vi "Dashboard Main.vi"() -> ()   [LabVIEW 2012]
uses:
  NonDriveDisplayPanel.ctl
  firstRoboticsCode2012/Snake Game/Snake/xyplot.ctl
  TestProject/Dashboard Datatype.ctl
  TestProject/All_Commands.ctl
  TestProject/Cirular Shooter/circular_shooter_commands.ctl
  TestProject/Climber/Climber_Commands.ctl
  TestProject/All_Outputs.ctl
  TestProject/Cirular Shooter/Shooter_Outputs.ctl
  TestProject/Climber/Climber_Outputs.ctl
  TestProject/All_Sensor_Readings.ctl
  TestProject/Climber/climber_sensor_readings.ctl
  TestProject/Cirular Shooter/Shooter_inputs.ctl
  TestProject/Field Drive/Field_Drive_out.ctl
  TestProject/Joystick_Inputs.ctl
  <vilib>/Rock Robotics/WPI/Joystick/WPI_JoystickButtonState.ctl
  <vilib>/Utility/config.llb/Read Key (String).vi
  <vilib>/Utility/config.llb/Read Key (I32).vi
  <vilib>/Utility/config.llb/NI_LVConfig.lvlib
  <vilib>/vision/NI_Vision_Development_Module.lvlib
panel:
  out "Status":T1(ring)
  in  "Force Hide Snake":bool
  out "direction1":dbl
  in  "Done":bool
  in  "Difficulty":dbl(ring)=15.0 items=["Applications Engineer"=15.0, "Insane"=30.0, "Advanced"=50.0, "Intermediate"=85.0, "Noobie"=125.0]
  in  "Max Apples":i32=10
  out "Score 1":i32
  out "XY Graph":cluster{i32[], i32[]}[](graph)=[{[1000, 990, 980, 970, 960, 950, 940, 930, 920, 910, 900, 890, 880, 870, 860, 850, 840, 830, 820, 810, 800, 790, 780, 770, 760, 750, 740, 730, 720, 710, 700, 690, 680, 670, 660, 650], [500, 500, 500, 500, 500, 500, 500, 500, 500, 500, 500, 500, 500, 500, 500, 500, 500, 500, 500, 500, 500, 500, 500, 500, 500, 500, 500, 500, 500, 500, 500, 500, 500, 500, 500, 500]}, {[-10, 0, 10, 20, 30, 40, 50, 60, 70, 80, 90, 100, 110, 120, 130, 140, 150, 160, 170, 180, 190, 200, 210, 220, 230, 240, 250, 260, 270, 280, 290, 300, 310, 320, 330, 340], [500, 500, 500, 500, 500, 500, 500, 500, 500, 500, 500, 500, 500, 500, 500, 500, 500, 500, 500, 500, 500, 500, 500, 500, 500, 500, 500, 500, 500, 500, 500, 500, 500, 500, 500, 500]}, {[927, 615, 797, 523, 657, 721, 657, 632, 338, 606], [396, 821, 872, 400, 891, 885, 928, 521, 351, 556]}] caption="449"
  out "Score 2":i32
  out "direction2":dbl=2.0
  in  "Add To Score":bool=TRUE
  out "Mechanism Display":T2 {"Current Shooter VBus" scale=0.0..1.0; "Shooter Angle" scale=-10.0..40.0}
  out "Drive Slow Mode":bool
  in  "Running w/ Camera?":bool=TRUE
  out "Camera Image":T3(plugin-control)
  out "Master Caution\nYou mess with the panda,\nsomebody gonna get hurt\nreal bad":bool
  out "Right Joystick":cluster{dbl[], dbl[]}(graph)
  out "Left Joystick":cluster{dbl[], dbl[]}(graph)
  out "BRight":dbl(slide) scale=0.0..1.0
  out "BLeft":dbl(slide) scale=0.0..1.0
  out "FRight":dbl(slide) scale=0.0..1.0
  out "FLeft":dbl(slide) scale=0.0..1.0
  out "Battery Value":dbl(slide) scale=0.0..14.0 scale format="%#_2e"
  out "Battery":sgl(graph)
  out "Mode":T4(ring)=enum."Auto Disabled"
  out "Camera IP":string
  out "Robot IP":string
  # "Wheel Power Requested"
  # "Robot IP:"
  # "Front"
  # "Back"
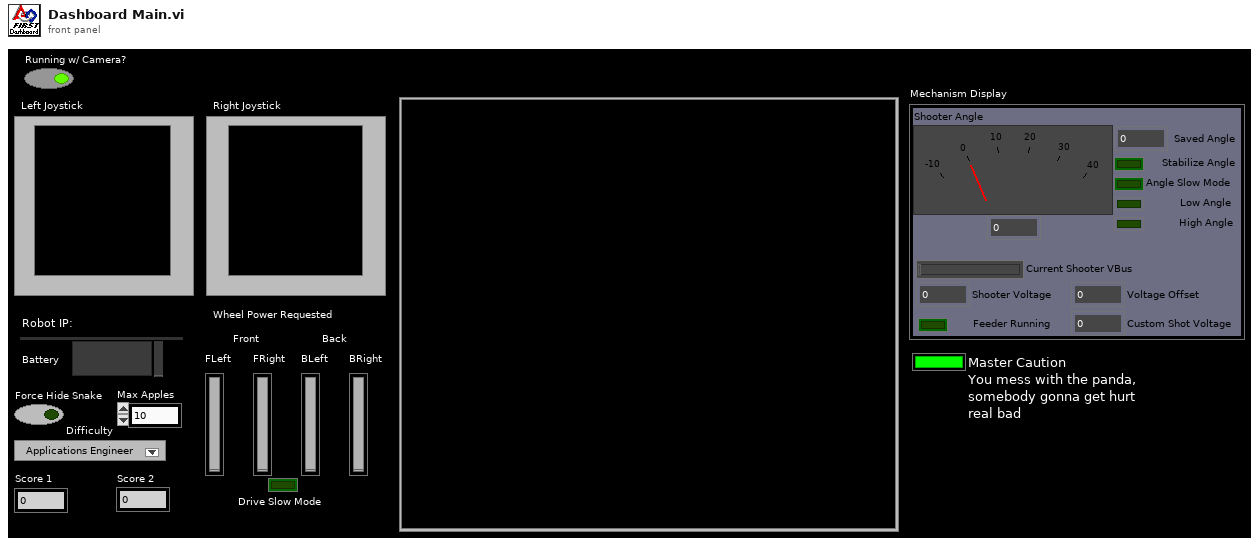
[diagram p1: front panel]
types:
  T1 = enum8{"Disconnected", "E-Stop", "Disabled", "Enabled"}
  T2 = typedef "NonDriveDisplayPanel.ctl" = cluster{"Shooter Angle":dbl, "Current Shooter VBus":dbl, "Shooter Voltage":dbl, "Feeder Running":bool, "Saved Angle":dbl, "Stabilize Angle":bool, "Voltage Offset":dbl, "Custom Shot Voltage":dbl, "Angle Slow Mode":bool, "Low Angle ":bool, "High Angle":bool}
  T3 = typedef "IMAQ Image.ctl" = refnum<image>
  T4 = enum8{"Tele-Op Disabled", "Tele-Op Enabled", "Auto Disabled", "Auto Enabled", "Test Disabled", "Test Enabled", ""}
  T5 = typedef "Image Type" = u32
  T6 = typedef "Dashboard Datatype.ctl" = cluster{"All Driver Commands":T7, "All_Outputs":T10, "All_Sensor_Readings":T13, "Joystick_Inputs ":T17}
  T7 = typedef "All_Commands.ctl" = cluster{"Circular Shooter Commands":T8, "Drive Command Inputs":cluster{"Strafe":dbl, "Forward/Backward":dbl, "Rotation":dbl, "Drive Slow Toggle":bool}, "Climber_Commands":T9}
  T8 = typedef "circular_shooter_commands.ctl" = cluster{"Shoot?":bool, "Angle Change":dbl, "Close Shot":bool, "Far Shot":bool, "Stabilize Angle ":bool, "Offset":dbl, "Custom Shot":bool, "Custom Shot Voltage":dbl, "Low Angle":bool, "High Angle":bool, "Angle Slow Mode":bool, "Dejam":bool, "Save Angle":bool, "Saved Preset Angle":bool}
  T9 = typedef "Climber_Commands.ctl" = cluster{"Assist":dbl}
  T10 = typedef "All_Outputs.ctl" = cluster{"Drive Outputs":cluster{"Front Left\nSpeed":dbl, "Back Left\nSpeed":dbl, "Front Right\nSpeed":dbl, "Back Right\nSpeed":dbl}, "Shooter_Outputs":T11, "Climber_Outputs":T12}
  T11 = typedef "Shooter_Outputs.ctl" = cluster{"Feeder_Motor_Voltage":dbl, "Output Voltage":dbl, "Overloaded":bool, "Variable_Angle_Voltage":dbl, "Saved Angle":dbl}
  T12 = typedef "Climber_Outputs.ctl" = cluster{"Assist Voltage":dbl}
  T13 = typedef "All_Sensor_Readings.ctl" = cluster{"Climber Inputs":T14, "Drive Sensor Readings":cluster{"Front Left\nSpeed":dbl, "Back Left\nSpeed":dbl, "Front Right\nSpeed":dbl, "Back Right\nSpeed":dbl}, "Shooter_Inputs":T15, "Field_Drive_Out\n":T16}
  T14 = typedef "climber_sensor_readings.ctl" = cluster{"Top Left Switch":bool, "Bottom Left Switch":bool, "Top Right Switch":bool, "Bottom Right Switch":bool}
  T15 = typedef "Shooter_inputs.ctl" = cluster{"Bus Voltage":dbl, "Output Percent VBus":dbl, "Shooter Elevation Angle":dbl, "FeederPosition":bool}
  T16 = typedef "Field_Drive_out.ctl" = cluster{"XPos":dbl, "Ypos":dbl, "XVel":dbl, "YVel":dbl, "Heading":dbl, "AngularVel":dbl, "F_XPos":dbl, "F_Ypos":dbl, "F_Angle":dbl}
  T17 = typedef "Joystick_Inputs.ctl" = cluster{"Joystick 1":cluster{"Axes":cluster{"axis 1 (x)":dbl, "axis 2 (y)":dbl, "axis 3 (throttle)":dbl, "axis 4":dbl, "axis 5":dbl, "axis 6":dbl}, "Buttons":T18}, "Joystick 2":cluster{"Axes":cluster{"axis 1 (x)":dbl, "axis 2 (y)":dbl, "axis 3 (throttle)":dbl, "axis 4":dbl, "axis 5":dbl, "axis 6":dbl}, "Buttons":T18}, "Joystick 3":cluster{"Axes":cluster{"axis 1 (x)":dbl, "axis 2 (y)":dbl, "axis 3 (throttle)":dbl, "axis 4":dbl, "axis 5":dbl, "axis 6":dbl}, "Buttons":T18}, "Joystick 4":cluster{"Axes":cluster{"axis 1 (x)":dbl, "axis 2 (y)":dbl, "axis 3 (throttle)":dbl, "axis 4":dbl, "axis 5":dbl, "axis 6":dbl}, "Buttons":T18}}
  T18 = typedef "WPI_JoystickButtonState.ctl" = cluster{"Button 1":bool, "Button 2":bool, "Button 3":bool, "Button 4":bool, "Button 5":bool, "Button 6":bool, "Button 7":bool, "Button 8":bool, "Button 9":bool, "Button 10":bool, "Button 11":bool, "Button 12":bool}
  T19 = cluster{"Competition mode":bool, "Robot Link":bool, "Autonomous":bool, "Enabled":bool, "E-Stop":bool, "Simulated":bool, "TestMode":bool, "Docked Window":bool}
  T20 = typedef "LVRectTypeDef.ctl" = cluster{"Left":i16, "Top":i16, "Right":i16, "Bottom":i16}
  T21 = typedef "NI_LVConfig.lvlib/Config Data RefNum.ctl" = refnum<k1>
  T22 = typedef "xyplot.ctl" = cluster{"X":i32[], "Y":i32[]}
  T23 = typedef "eventvkey.ctl" = enum16{"ASCII", "Enter", "Return", "Shift", "Ctrl", "Alt", "Cmd", "Opt", "Caps", "NumLock", "Clear", "Break", "Up", "Down", "Left", "Right", "Insert", "Delete", "Home", "End", "PageUp", "PageDown", "Escape", "Help", "Pause", "ScrollLock", "F1", "F2", "F3", "F4", "F5", "F6", "F7", "F8", "F9", "F10", "F11", "F12", "F13", "F14", "F15", "F16", "F17", "F18", "F19", "F20", "F21", "F22", "F23", "F24", "Play", "VolumeUp", "VolumeDown", "Mute", "Two Byte Char"}
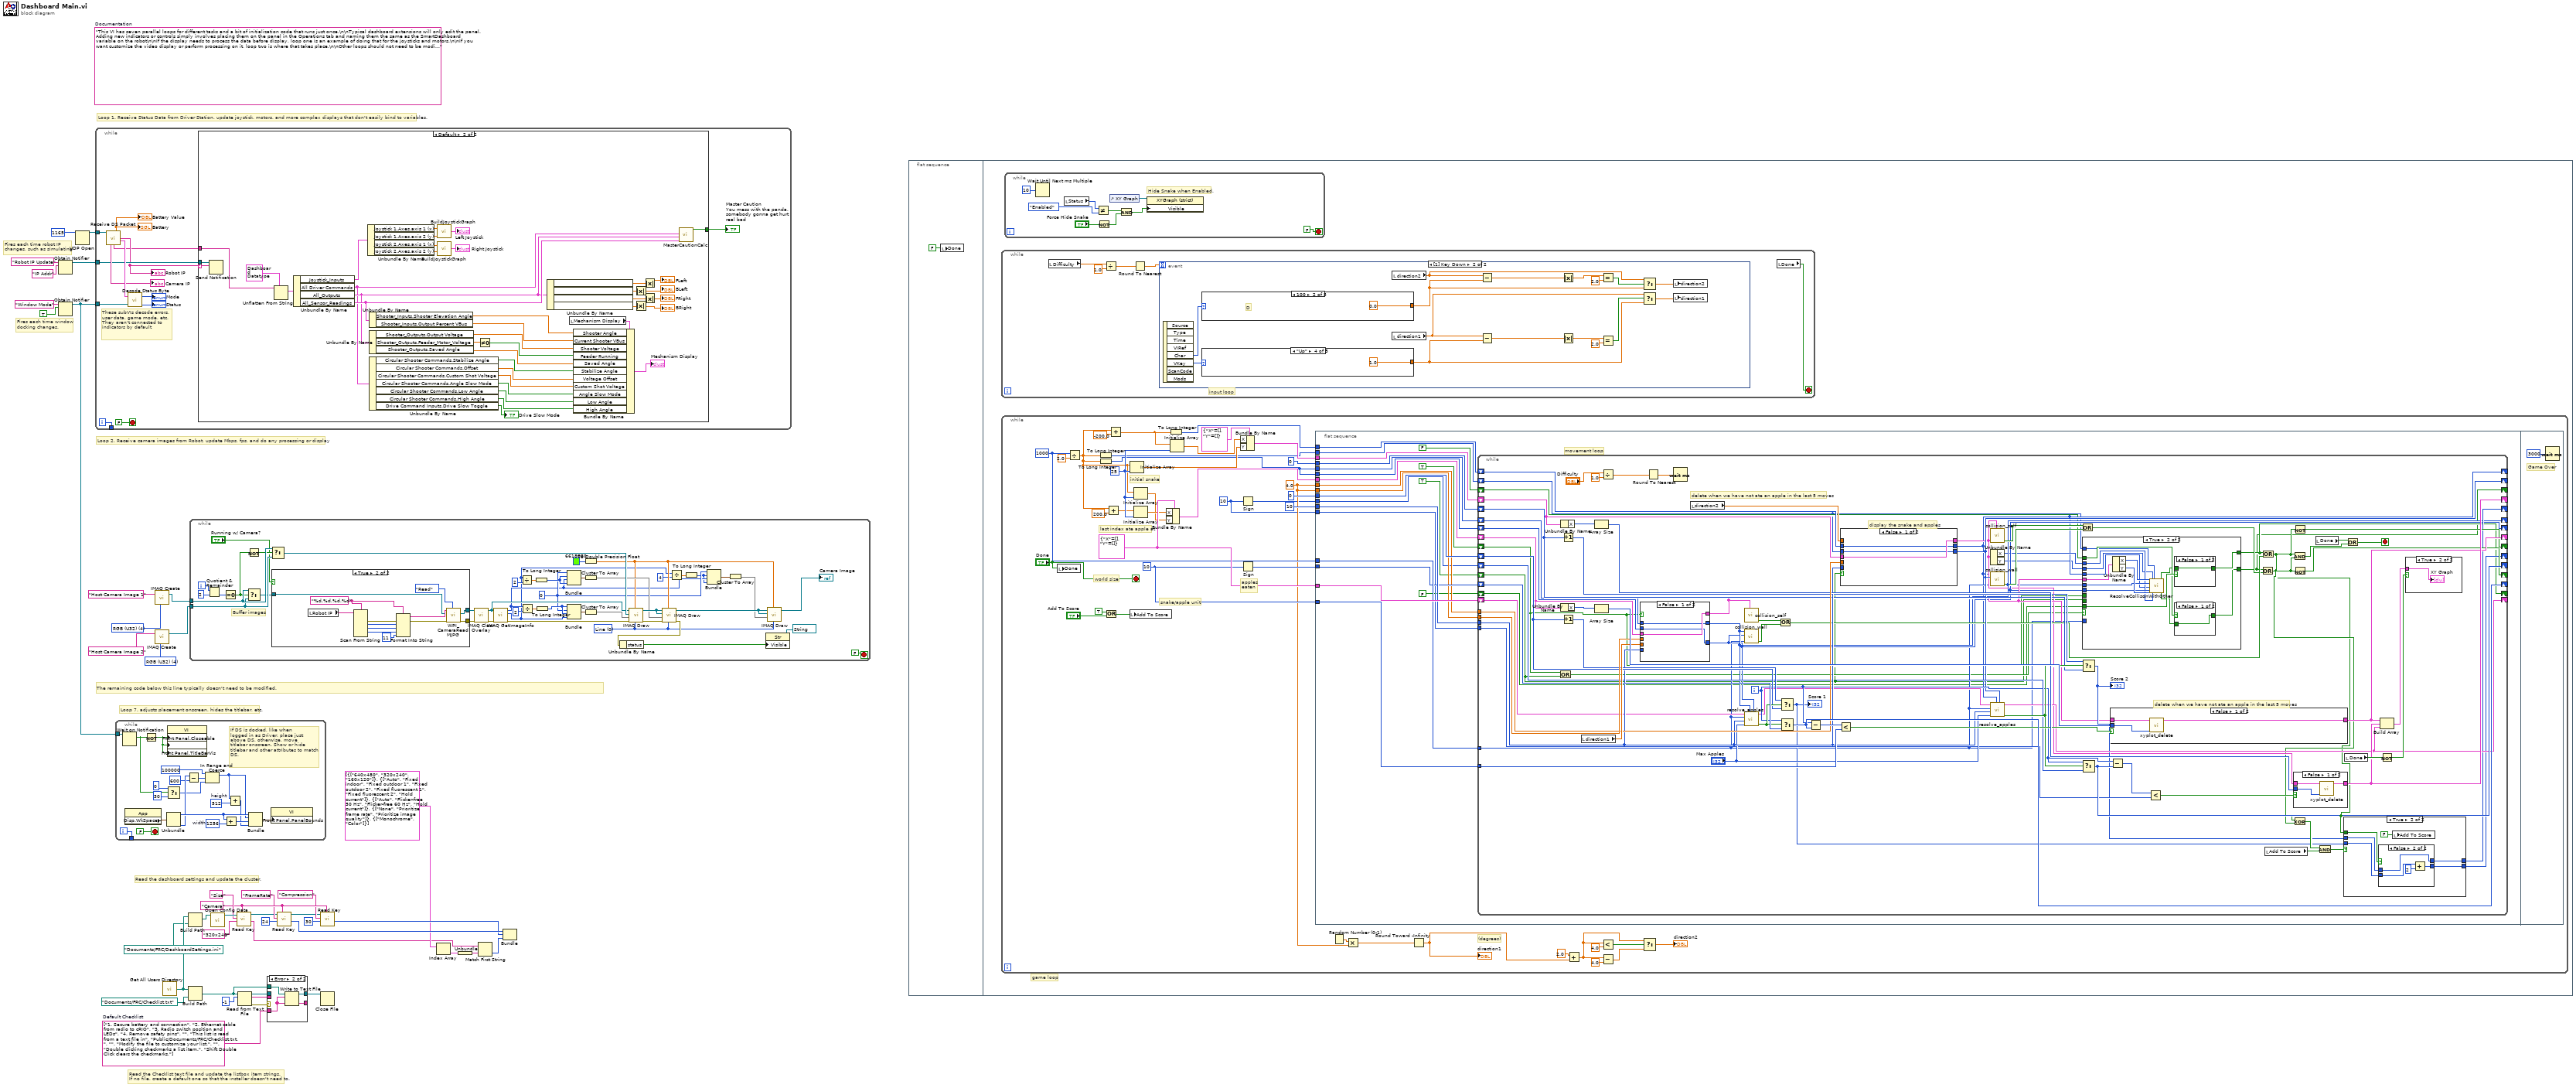
[diagram p0: block diagram]
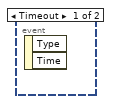
[diagram p2: hidden frame]
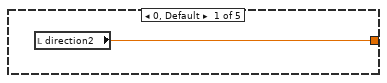
[diagram p3: hidden frame]
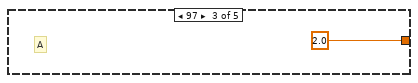
[diagram p4: hidden frame]
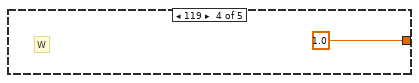
[diagram p5: hidden frame]
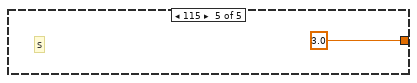
[diagram p6: hidden frame]
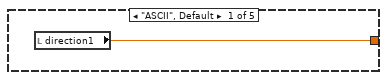
[diagram p7: hidden frame]
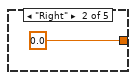
[diagram p8: hidden frame]
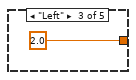
[diagram p9: hidden frame]
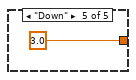
[diagram p10: hidden frame]
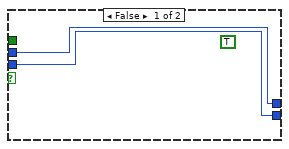
[diagram p16: hidden frame]
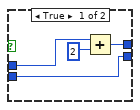
[diagram p17: hidden frame]
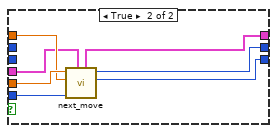
[diagram p18: hidden frame]
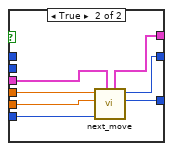
[diagram p19: hidden frame]
diagram:
  (unwired) "320x240"
  w3 = T5 4 items=["Grayscale (U8)", "Grayscale (I16)", "Grayscale (SGL)", "Complex (CSG)", "RGB (U32)", "HSL (U32)", "RGB (U64)", "Grayscale (U16)"] ("Image Type")
  w6 = T5 4 items=["Grayscale (U8)", "Grayscale (I16)", "Grayscale (SGL)", "Complex (CSG)", "RGB (U32)", "HSL (U32)", "RGB (U64)"] ("Image Type")
  w23 = "Camera"
  w29 = string[] ["1. Secure battery and connection", "2. Ethernet cable from radio to cRIO", "3. Radio switch position and LEDs", "4. Remove safety pins", "", "This list is read from a text file in", "Public/Documents/FRC/Checklist.txt.", "", "Modify the file to customize your list.", "", "Double clicking checkmarks a list item.", "Shift Double Click clears the checkmarks."]  # Default Checklist
  (unwired) "This VI has seven parallel loops for different tasks and a bit of initialization code that runs just once.\n\nTypical dashboard extensions will only edit the panel. Adding new indicators or controls simply involves placing them on the panel in the Operations tab and naming them the same as the SmartDashboard variable on the robot\n\nIf the display needs to process the data before display, loop one is an example of doing that for the joysticks and motors.\n\nIf you want customize the video display or perform processing on it, loop two is where that takes place.\n\nOther loops should not need to be modified. They are pretty standard, and document the task they perform."  # Documentation
  # "Fires each time robot IP\nchanges, such as simulating"
  # "Fires each time window\ndocking changes."
  # "Read the Checklist text file and update the listbox item strings.\nIf no file, create a default one so that the installer doesn't need to."
  # "The remaining code below this line typically doesn't need to be modified."
  # "Read the dashboard settings and update the cluster."
  # "Loop 7. adjusts placement onscreen, hides the titlebar, etc."
  # "Loop 1. Receive Status Data from Driver Station, update joystick, motors, and more complex displays that don't easily bind to variables."
  # "Loop 2. Receive camera images from Robot, update Mbps, fps, and do any processing or display"
  n1 = Obtain Notifier(name (unnamed)="Robot IP Update", notification data type="IP Addr" ("name (unnamed)")) -> (notifier out=w38:refnum<notifier>)  [unwired: 2 in, 2 out]
  n2 = Obtain Notifier(name (unnamed)="Window Mode", notification data type=TRUE) -> (notifier out=w33:refnum<notifier>)  [unwired: 2 in, 2 out]
  n3 = UDP Open(11:u16 1165 ("port")) -> (port=w41:refnum<k16>)  [unwired: 2 in, 4 out]
  n4 = while {
    tunnel: w41 -> [w53]
    tunnel: w38 -> [w47]
    tunnel: w33 -> [w51]
    tunnel: [w48] -> _
    i -> [w48]
    stop <- FALSE stop-if-true
    # "These subVIs decode errors, user data, game mode, etc.\nThey aren't connected to indicators by default"
    n5 = call "Receive DS Packet.vi"("Recv Socket"=w53) -> ("Battery"=→"Battery" →"Battery Value":sgl, "Robot IP Address"=w46:string, "Status"=w54:T19, "Camera IP Address"=→"Camera IP":string, "Low Priority User Data"=w43:string)  [unwired: 1 in, 9 out]
    "Robot IP" <- w46
    n6 = call "Decode Status Byte.vi"("Window Mode Notifier"=w51, "Status"=w54) -> ("Status"=→"Status":T1, "Mode"=→"Mode":T4)
    n7 = case shown="Default" w46 {
      selector: w46 -> [_ w94]
      tunnel: w47 -> [_ w95]
      tunnel: [TRUE w77] -> w45
      tunnel: w43 -> [_ w59]
      frame "0.0.0.0" {
        # "Robot not responding, don't poll the variables"
      }
      frame Default {
        n8 = Send Notification(notification=w94, notifier=w95) -> ()  [unwired: 1 in, 2 out]
        n9 = Unflatten From String(type=T6 {"All Driver Commands"={"Circular Shooter Commands"={"Shoot?"=FALSE, "Angle Change"=0.0, "Close Shot"=FALSE, "Far Shot"=FALSE, "Stabilize Angle "=FALSE, "Offset"=0.0, "Custom Shot"=FALSE, "Custom Shot Voltage"=0.0, "Low Angle"=FALSE, "High Angle"=FALSE, "Angle Slow Mode"=FALSE, "Dejam"=FALSE, "Save Angle"=FALSE, "Saved Preset Angle"=FALSE}, "Drive Command Inputs"={"Strafe"=0.0, "Forward/Backward"=0.0, "Rotation"=0.0, "Drive Slow Toggle"=FALSE}, "Climber_Commands"={"Assist"=0.0}}, "All_Outputs"={"Drive Outputs"={"Front Left\nSpeed"=0.0, "Back Left\nSpeed"=0.0, "Front Right\nSpeed"=0.0, "Back Right\nSpeed"=0.0}, "Shooter_Outputs"={"Feeder_Motor_Voltage"=0.0, "Output Voltage"=0.0, "Overloaded"=FALSE, "Variable_Angle_Voltage"=0.0, "Saved Angle"=0.0}, "Climber_Outputs"={"Assist Voltage"=0.0}}, "All_Sensor_Readings"={"Climber Inputs"={"Top Left Switch"=FALSE, "Bottom Left Switch"=FALSE, "Top Right Switch"=FALSE, "Bottom Right Switch"=FALSE}, "Drive Sensor Readings"={"Front Left\nSpeed"=0.0, "Back Left\nSpeed"=0.0, "Front Right\nSpeed"=0.0, "Back Right\nSpeed"=0.0}, "Shooter_Inputs"={"Bus Voltage"=0.0, "Output Percent VBus"=0.0, "Shooter Elevation Angle"=0.0, "FeederPosition"=FALSE}, "Field_Drive_Out\n"={"XPos"=0.0, "Ypos"=0.0, "XVel"=0.0, "YVel"=0.0, "Heading"=0.0, "AngularVel"=0.0, "F_XPos"=0.0, "F_Ypos"=0.0, "F_Angle"=0.0}}, "Joystick_Inputs "={"Joystick 1"={"Axes"={"axis 1 (x)"=0.0, "axis 2 (y)"=0.0, "axis 3 (throttle)"=0.0, "axis 4"=0.0, "axis 5"=0.0, "axis 6"=0.0}, "Buttons"={"Button 1"=FALSE, "Button 2"=FALSE, "Button 3"=FALSE, "Button 4"=FALSE, "Button 5"=FALSE, "Button 6"=FALSE, "Button 7"=FALSE, "Button 8"=FALSE, "Button 9"=FALSE, "Button 10"=FALSE, "Button 11"=FALSE, "Button 12"=FALSE}}, "Joystick 2"={"Axes"={"axis 1 (x)"=0.0, "axis 2 (y)"=0.0, "axis 3 (throttle)"=0.0, "axis 4"=0.0, "axis 5"=0.0, "axis 6"=0.0}, "Buttons"={"Button 1"=FALSE, "Button 2"=FALSE, "Button 3"=FALSE, "Button 4"=FALSE, "Button 5"=FALSE, "Button 6"=FALSE, "Button 7"=FALSE, "Button 8"=FALSE, "Button 9"=FALSE, "Button 10"=FALSE, "Button 11"=FALSE, "Button 12"=FALSE}}, "Joystick 3"={"Axes"={"axis 1 (x)"=0.0, "axis 2 (y)"=0.0, "axis 3 (throttle)"=0.0, "axis 4"=0.0, "axis 5"=0.0, "axis 6"=0.0}, "Buttons"={"Button 1"=FALSE, "Button 2"=FALSE, "Button 3"=FALSE, "Button 4"=FALSE, "Button 5"=FALSE, "Button 6"=FALSE, "Button 7"=FALSE, "Button 8"=FALSE, "Button 9"=FALSE, "Button 10"=FALSE, "Button 11"=FALSE, "Button 12"=FALSE}}, "Joystick 4"={"Axes"={"axis 1 (x)"=0.0, "axis 2 (y)"=0.0, "axis 3 (throttle)"=0.0, "axis 4"=0.0, "axis 5"=0.0, "axis 6"=0.0}, "Buttons"={"Button 1"=FALSE, "Button 2"=FALSE, "Button 3"=FALSE, "Button 4"=FALSE, "Button 5"=FALSE, "Button 6"=FALSE, "Button 7"=FALSE, "Button 8"=FALSE, "Button 9"=FALSE, "Button 10"=FALSE, "Button 11"=FALSE, "Button 12"=FALSE}}}} ("Dashboard Data"), binary string=w59) -> (value=w93:T6)  [unwired: 3 in, 2 out]
        n10 = Unbundle By Name(w93) -> ("Joystick_Inputs"=w84:T17, "All Driver Commands"=w73:T7, "All_Outputs"=w75:T10, "All_Sensor_Readings"=w76:T13)
        n11 = Unbundle By Name(w84) -> ("Joystick 1.Axes.axis 1 (x)"=w81:dbl, "Joystick 1.Axes.axis 2 (y)"=w80:dbl, "Joystick 2.Axes.axis 1 (x)"=w79:dbl, "Joystick 2.Axes.axis 2 (y)"=w78:dbl)
        n12 = Unbundle By Name(w76) -> ("Shooter_Inputs.Shooter Elevation Angle"=w57:dbl, "Shooter_Inputs.Output Percent VBus"=w70:dbl)
        n13 = Unbundle By Name(w75) -> ("Shooter_Outputs.Output Voltage"=w69:dbl, "Shooter_Outputs.Feeder_Motor_Voltage"=w74:dbl, "Shooter_Outputs.Saved Angle"=w67:dbl)
        n14 = Unbundle By Name(w73) -> ("Circular Shooter Commands.Stabilize Angle"=w66:bool, "Circular Shooter Commands.Offset"=w65:dbl, "Circular Shooter Commands.Custom Shot Voltage"=w64:dbl, "Circular Shooter Commands.Angle Slow Mode"=w63:bool, "Circular Shooter Commands.Low Angle"=w61:bool, "Circular Shooter Commands.High Angle"=w60:bool, "Drive Command Inputs.Drive Slow Toggle"=→"Drive Slow Mode":bool)
        n15 = call "BuildJoystickGraph.vi"("YAxis"=w80, "XAxis"=w81) -> ("Left Joystick"=→"Left Joystick":cluster{dbl[], dbl[]})
        n16 = call "BuildJoystickGraph.vi"("YAxis"=w78, "XAxis"=w79) -> ("Left Joystick"=→"Right Joystick":cluster{dbl[], dbl[]})
        n17 = Not Equal To 0?(x=w74) -> (x != 0?=w68:bool)
        n18 = Unbundle By Name(w75) -> ("Drive Outputs.Front Left\nSpeed"=w92:dbl, "Drive Outputs.Back Left\nSpeed"=w91:dbl, "Drive Outputs.Front Right\nSpeed"=w89:dbl, "Drive Outputs.Back Right\nSpeed"=w90:dbl)
        n19 = local read "Mechanism Display"() -> (w71:T2)
        n20 = Bundle By Name(cluster=w71, "Shooter Angle"=w57, "Current Shooter VBus"=w70, "Shooter Voltage"=w69, "Feeder Running"=w68, "Saved Angle"=w67, "Stabilize Angle"=w66, "Voltage Offset"=w65, "Custom Shot Voltage"=w64, "Angle Slow Mode"=w63, "Low Angle"=w61, "High Angle"=w60) -> (→"Mechanism Display":T2)
        n21 = Absolute Value(x=w91) -> (abs(x)=→"BLeft":dbl)
        n22 = Absolute Value(x=w90) -> (abs(x)=→"BRight":dbl)
        n23 = Absolute Value(x=w92) -> (abs(x)=→"FLeft":dbl)
        n24 = Absolute Value(x=w89) -> (abs(x)=→"FRight":dbl)
        n25 = call "MasterCautionCalc.vi"("All_Sensor_Readings"=w76, "All_Outputs"=w75, "All Driver Commands"=w73) -> ("Master Caution"=w77:bool)  [unwired: 8 in]
      }
    }
    "Master Caution\nYou mess with the panda,\nsomebody gonna get hurt\nreal bad" <- w45
  }
  n26 = while {
    tunnel: w33 -> [w114]
    tunnel: [w112] -> _
    i -> [w112]
    stop <- FALSE stop-if-true
    w104 = 1256  # width
    w107 = 512  # height
    # "If DS is docked, like when\nlogged in as Driver, place just\nabove DS, otherwise, move\ntitlebar onscreen. Show or hide\ntitlebar and other attributes to match\nDS."
    n27 = Wait on Notification(notifier=w114) -> (notification=w99:bool)  [unwired: 3 in, 3 out]
    n28 = property class="App"() -> ("Disp.WkSpace"=w110:T20)  [unwired: 2 in, 2 out]
    n29 = Not(x=w99) -> (.not. x?=w113:bool)
    n30 = Unbundle(w110) -> ("Left"=w108:i16, "Bottom"=w105:i16)  [unwired: 2 out]
    n31 = Select(t=0, s=w99, f=30) -> (s? t:f=w98:i32)
    n32 = property class="VI"("Front Panel.Closeable"=w113, "Front Panel.Minimizeable"=w113, "Front Panel.TitleBarVis"=w113) -> ()  [unwired: 2 in, 2 out]
    n33 = Subtract(x=w105, y=600) -> (x-y=w102:i32)
    n34 = In Range and Coerce(upper limit=100000, x=w102, lower limit=w98) -> (coerced(x)=w96:i32)  [unwired: 1 out]
    n35 = Add(x=w108, y=w104) -> (x+y=w109:i32)
    n36 = Add(x=w96, y=w107) -> (x+y=w106:i32)
    n37 = Bundle("Left"=w108, w96, w109, w106) -> (w111:cluster{"Left":i16, i32, i32, i32})  [unwired: 1 out]
    n38 = property class="VI"("Front Panel.PanelBounds"=w111) -> ()  [unwired: 2 in, 2 out]
  }
  n39 = call "IMAQ Create"("Image Name"="Host Camera Image 1", "Image Type"=w6) -> ("New Image"=w2:T3)  [unwired: 2 in, 2 out]
  n40 = call "IMAQ Create"("Image Name"="Host Camera Image 2", "Image Type"=w3) -> ("New Image"=w1:T3)  [unwired: 3 in, 1 out]
  n41 = call "Get All Users Directory.vi"() -> ("All User Path"=w28:path)
  n42 = Build Path(base path=w28, name or relative path=path "Documents/FRC/DashboardSettings.ini") -> (appended path=w27:path)
  n43 = Build Path(base path=w28, name or relative path=path "Documents/FRC/Checklist.txt") -> (appended path=w30:path)
  n44 = while {
    tunnel: w2 -> [w158]
    tunnel: w1 -> [w153]
    i -> [w157]
    stop <- FALSE stop-if-true
    w121 = 0
    w124 = u16 0 items=["Line", "Rectangle", "Oval"] ("Shape to draw")
    # "Buffer images"
    n45 = Quotient & Remainder(x=w157, y=2) -> (floor(x/y)=w155:i32)  [unwired: 1 out]
    n46 = Equal To 0?(x=w155) -> (x = 0?=w154:bool)
    n47 = Not(x=w154) -> (.not. x?=w144:bool)
    n48 = Select(t=w158, s=w154, f=w153) -> (s? t:f=w141:T3)
    n49 = Select(t=w158, s=w144, f=w153) -> (s? t:f=w143:T3)
    n50 = case shown="True" "Running w/ Camera?" {
      tunnel: w141 -> [w169 w172]
      tunnel: [w167 w170] -> w146
      tunnel: [w168 w171] -> w145
      frame False {
        n51 = Current VI's Path() -> (path=w166:path)
        n52 = Strip Path(path=w166) -> (stripped path=w165:path)  [unwired: 1 out]
        n53 = Strip Path(path=w165) -> (stripped path=w160:path)  [unwired: 1 out]
        n54 = Build Path(base path=w160, name or relative path="Vision") -> (appended path=w163:path)
        n55 = Build Path(base path=w163, name or relative path="Field1.jpg") -> (appended path=w161:path)
        n56 = call "IMAQ ReadFile"("File Path"=w161, "Image"=w169) -> ("error out"=w167:errorcluster, "Image Out"=w168:T3)  [unwired: 5 in, 3 out]
      }
      frame True {
        w176 = "%d.%d.%d.%d" ("format string")
        n57 = local read "Robot IP"() -> (w173:string)
        n58 = Scan From String(format string=w176, input string=w173) -> (error out=w179:errorcluster, output 1=w180:i32, output 2=w181:i32, output 3=w182:i32)  [unwired: 2 in, 7 out]
        n59 = Format Into String(format string=w176, error in=w179, w180, w181, w182, 11 ("IP Suffix:")) -> (resulting string=w178:string, error out=w177:errorcluster)  [unwired: 1 in]
        n60 = call <vilib>:"WPI_CameraRead MJPG.vi"("Operation"=enum16{"Read", "Reopen", "Close"}."Read", "error in"=w177, "Image"=w172, "address"=w178) -> ("error out"=w170:errorcluster, "Image Out"=w171:T3)  [unwired: 5 in, 1 out]
      }
    }
    n61 = call "IMAQ Clear Overlay"("error in (no error)"=w146, "Image"=w145) -> ("error out"=w139:errorcluster, "Image Out"=w140:T3)  [unwired: 8 in]
    n62 = call "IMAQ GetImageInfo"("error in (no error)"=w139, "Image"=w140) -> ("error out"=w147:errorcluster, "Y Resolution"=w119:i32, "X Resolution"=w120:i32)  [unwired: 2 in, 5 out]
    n63 = Divide(x=w119, y=2) -> (x/y=w130:dbl)
    n64 = Divide(x=w120, y=2) -> (x/y=w151:dbl)
    n65 = To Long Integer(number=w130) -> (32bit integer=w129:i32)
    n66 = To Long Integer(number=w151) -> (32bit integer=w150:i32)
    n67 = Bundle(w121, w129, "X Resolution"=w120, w129) -> (w133:cluster{i32, i32, "X Resolution":i32, i32})  [unwired: 1 in]
    n68 = Bundle(w150, w121, w150, "Y Resolution"=w119) -> (w149:cluster{i32, i32, i32, "Y Resolution":i32})  [unwired: 1 in]
    n69 = Cluster To Array(cluster=w133) -> (array=w132:i32[])
    n70 = Cluster To Array(cluster=w149) -> (array=w148:i32[])
    n71 = To Double Precision Float(number=u32 6618880) -> (double precision float=w127:dbl)
    n72 = call "IMAQ Draw"("Shape to draw"=w124, "Pixel Color"=w127, "error in (no error)"=w147, "Coordinates"=w148, "Image Dst"=w143, "Image Src"=w140) -> ("error out"=w136:errorcluster, "Image Dst Out"=w134:T3)  [unwired: 4 in]
    n73 = call "IMAQ Draw"("Shape to draw"=w124, "Pixel Color"=w127, "error in (no error)"=w136, "Coordinates"=w132, "Image Dst"=w134, "Image Src"=w134) -> ("error out"=w135:errorcluster, "Image Dst Out"=w125:T3)  [unwired: 4 in]
    n74 = Unbundle By Name(w135) -> ("status"=w138:bool)
    n75 = Divide(x=w119, y=4) -> (x/y=w117:dbl)
    n76 = To Long Integer(number=w117) -> (32bit integer=w116:i32)
    n77 = Bundle(w121, w116, "X Resolution"=w120, w116) -> (w122:cluster{i32, i32, "X Resolution":i32, i32})  [unwired: 1 in]
    n78 = Cluster To Array(cluster=w122) -> (array=w123:i32[])
    n79 = property on="Property Node" class="Str"(reference=refnum<vi> refnum, "Visible"=w138) -> ()  [unwired: 1 in, 2 out]
    n80 = call "IMAQ Draw"("Shape to draw"=w124, "Pixel Color"=w127, "Coordinates"=w123, "Image Dst"=w125, "Image Src"=w125) -> ("Image Dst Out"=→"Camera Image":T3)  [unwired: 5 in, 1 out]
  }
  n81 = call <vilib>:"Open Config Data.vi"("configuration file path"=w27) -> ("refnum"=w26:T21)  [unwired: 8 in, 2 out]
  n82 = call-poly <vilib>:"Read Key.vi"("section"=w23, "default value"="320x240", "key"="Size", "refnum"=w26) -> ("value"=w13:string, "refnum out"=w8:T21)  [unwired: 2 in, 4 out]
  n83 = Read from Text File(file (use dialog)=w30, count=-1 ("timeout ms (25000)")) -> (refnum out=w10:refnum<file>, text=w31:string[], error out=w32:errorcluster)  [unwired: 2 in, 1 out]
  n84 = case shown="Error" w32 {
    tunnel: w31 -> [w184 _]
    tunnel: [w184 w186] -> _
    tunnel: w29 -> [_ w186]
    tunnel: w30 -> [_ w187]
    tunnel: [w183 w185] -> w9
    tunnel: w10 -> [w183 _]
    frame No Error {
    }
    frame Error {
      n85 = Write to Text File(file (use dialog)=w187, text=w186) -> (refnum out=w185:refnum<file>)  [unwired: 2 in, 2 out]
    }
  }
  n86 = call-poly <vilib>:"Read Key.vi"("section"=w23, "default value"=24, "key"="FrameRate", "refnum"=w8) -> ("value"=w18:i32, "refnum out"=w7:T21)  [unwired: 1 in, 5 out]
  n87 = Close File(refnum=w9) -> ()  [unwired: 1 in, 2 out]
  n88 = call-poly <vilib>:"Read Key.vi"("section"=w23, "default value"=30, "key"="Compression", "refnum"=w7) -> ("value"=w17:i32)  [unwired: 1 in, 6 out]
  n89 = Index Array(array=cluster{string[]}[] [{["640x480", "320x240", "160x120"]}, {["Auto", "Fixed indoor", "Fixed outdoor 1", "Fixed outdoor 2", "Fixed fluorescent 1", "Fixed fluorescent 2", "Hold current"]}, {["Auto", "Flicker-free 50 Hz", "Flicker-free 60 Hz", "Hold current"]}, {["None", "Prioritize frame rate", "Prioritize image quality"]}, {["Monochrome", "Color"]}]) -> (element=w16:cluster{string[]})  [unwired: 1 in]
  n90 = Unbundle(w16) -> (w14:string[])
  n91 = Match First String(2:w14, 3:w13) -> (0:w12:i32)  [unwired: 1 out]
  n92 = Bundle("value"=w18, "value"=w17, "index"=w12) -> ()  [unwired: 2 out]
  n93 = flat-sequence {
    frame #0 {
      n94 = local write "Done"(FALSE ("Done")) -> ()
    }
    frame #1 {
      # "game loop"
      n95 = while {
        stop <- w201 stop-if-true
        # "input loop"
        n96 = local read "Difficulty"() -> (w202:dbl)
        n97 = Divide(x=w202, y=1.0) -> (x/y=w200:dbl)
        n98 = Round To Nearest(number=w200) -> (nearest integer value=w198:dbl)
        n99 = event shown="[1] Key Down" {
          selector: _ -> [_ _]
          dyn-events: _ -> [_ _]
          timeout: w198 -> [_ _]
          event Timeout {
            n100 = event-data() -> ()  [unwired: 1 in, 2 out]
          }
          event Key Down {
            n101 = event-data() -> ("Char"=w204:i16, "VKey"=w218:T23)  [unwired: 1 in, 6 out]
            n102 = case shown="100" w204 {
              tunnel: [w219 0.0 ("direction2") 2.0 ("direction2") 1.0 ("direction2") 3.0 ("direction2")] -> w203
              frame 0, Default {
                n103 = local read "direction2"() -> (w219:dbl)
              }
              frame 100 {
                # "D"
              }
              frame 97 {
                # "A"
              }
              frame 119 {
                # "W"
              }
              frame 115 {
                # "S"
              }
            }
            n104 = case shown="\"Up\"" w218 {
              tunnel: [w224 0.0 ("y") 2.0 ("y") 1.0 ("y") 3.0 ("y")] -> w213
              frame "ASCII", Default {
                n105 = local read "direction1"() -> (w224:dbl)
              }
              frame "Right" {
              }
              frame "Left" {
              }
              frame "Up" {
              }
              frame "Down" {
              }
            }
            n106 = local read "direction2"() -> (w205:dbl)
            n107 = local read "direction1"() -> (w214:dbl)
            n108 = Subtract(x=w205, y=w203) -> (x-y=w210:dbl)
            n109 = Subtract(x=w214, y=w213) -> (x-y=w217:dbl)
            n110 = Absolute Value(x=w210) -> (abs(x)=w209:dbl)
            n111 = Absolute Value(x=w217) -> (abs(x)=w216:dbl)
            n112 = Equal?(x=w209, y=2.0) -> (x = y?=w208:bool)
            n113 = Equal?(x=w216, y=2.0) -> (x = y?=w215:bool)
            n114 = Select(t=w205, s=w208, f=w203) -> (s? t:f=w206:dbl)
            n115 = Select(t=w214, s=w215, f=w213) -> (s? t:f=w211:dbl)
            n116 = local write "direction2"(w206) -> ()
            n117 = local write "direction1"(w211) -> ()
          }
        }
        n118 = local read "Done"() -> (w201:bool)
      }
      n119 = while {
        stop <- "Done" stop-if-true
        w247 = 10
        w252 = 4.0
        w259 = 10
        w255 = 25 ("y")
        w268 = T22 {"X"=[], "Y"=[]} ("XY Plot")
        w264 = 1000 ("y")
        # "apples\neaten"
        # "last index ate apple at"
        # "world size"
        # "snake/apple unit"
        # "(degrees)"
        # "initial snake"
        n120 = local write "Done"("Done") -> ()
        n121 = Divide(x=w264, y=2.0) -> (x/y=w231:dbl)
        n122 = To Long Integer(number=w231) -> (32bit integer=w229:i32)
        n123 = To Long Integer(number=w231) -> (32bit integer=w239:i32)
        n124 = Or(x=TRUE, y="Add To Score") -> (x .or. y?=w237:bool)
        n125 = Add(x=w231, y=200.0) -> (x+y=w235:dbl)
        n126 = Add(x=w231, y=-200.0) -> (x+y=w232:dbl)
        n127 = Initialize Array(w231, w255) -> (w253:dbl[])
        n128 = local write "Add To Score"(w237) -> ()
        n129 = Initialize Array(w231, w255) -> (w262:dbl[])
        n130 = Initialize Array(w235, w255) -> (w263:dbl[])
        n131 = Bundle By Name(cluster=w268, "X"=w263, "Y"=w262) -> (w267:T22)
        n132 = To Long Integer(number=w232) -> (32bit integer=w230:i32)
        n133 = Initialize Array(w232, w255) -> (w254:dbl[])
        n134 = Bundle By Name(cluster=T22 {"X"=[], "Y"=[]} ("XY Plot"), "X"=w254, "Y"=w253) -> (w251:T22)
        n135 = Sign(1:w247) -> (0:w248:i32)
        n136 = Sign(1:w259) -> (0:w260:i32)
        n137 = flat-sequence {
          tunnel: w268 -> [w290]
          tunnel: w267 -> [w289]
          tunnel: w264 -> [w288]
          tunnel: 10 -> [w287]
          tunnel: w260 -> [w286]
          tunnel: w259 -> [w285]
          tunnel: 0 -> [w284]
          tunnel: w252 -> [w283]
          tunnel: w252 -> [w282]
          tunnel: w251 -> [w281]
          tunnel: 0 -> [w280]
          tunnel: w248 -> [w279]
          tunnel: w247 -> [w278]
          tunnel: w239 -> [w275]
          tunnel: w239 -> [w274]
          tunnel: w230 -> [w273]
          tunnel: w229 -> [w272]
          frame #0 {
            # "movement loop"
            n138 = while {
              shift-right: [w326] -> _
              shift-left: w289 -> [w365]
              shift-right: [w325] -> _
              shift-left: w290 -> [w335]
              tunnel: w287 -> [w340]
              tunnel: w288 -> [w303]
              tunnel: w283 -> [w368]
              shift-right: [w361] -> _
              shift-left: w286 -> [w364]
              tunnel: w285 -> [w362]
              shift-right: [w311] -> _
              shift-left: w284 -> [w359]
              tunnel: w282 -> [w349]
              shift-right: [w327] -> _
              shift-left: w281 -> [w347]
              shift-right: [w333] -> _
              shift-left: w279 -> [w336]
              shift-right: [w310] -> _
              shift-left: w280 -> [w337]
              tunnel: w278 -> [w330]
              shift-right: [w323] -> _
              shift-left: TRUE -> [w297]
              shift-right: [w322] -> _
              shift-left: TRUE -> [w296]
              shift-right: [w307] -> _
              shift-left: w275 -> [w320]
              shift-right: [w306] -> _
              shift-left: w274 -> [w321]
              shift-right: [w302] -> _
              shift-left: w273 -> [w319]
              shift-right: [w318] -> _
              shift-left: w272 -> [w291]
              shift-right: [w295] -> _
              shift-left: FALSE ("Snake 1 Died") -> [w294]
              shift-right: [w293] -> _
              shift-left: FALSE ("Snake 2 Died") -> [w292]
              i -> [w332]
              stop <- w354 stop-if-true
              # "delete when we have not ate an apple in the last 5 moves"
              # "display the snake and apples"
              # "delete when we have not ate an apple in the last 5 moves"
              n139 = Or(x=w297, y=w296) -> (x .or. y?=w298:bool)
              n140 = Unbundle By Name(w347) -> ("X"=w346:i32[])
              n141 = Unbundle By Name(w365) -> ("X"=w366:i32[])
              n142 = Increment(x=w337) -> (x+1=w338:i32)
              n143 = Increment(x=w359) -> (x+1=w358:i32)
              n144 = local read "direction1"() -> (w367:dbl)
              n145 = Array Size(array=w346) -> (size(s)=w345:i32)
              n146 = Array Size(array=w366) -> (size(s)=w371:i32)
              n147 = Divide(x="Difficulty", y=1.0) -> (x/y=w351:dbl)
              n148 = case shown="False" w297 {
                tunnel: w368 -> [_ w436]
                tunnel: w367 -> [_ w435]
                tunnel: [w429 w434] -> w308
                tunnel: [w427 w433] -> w307
                tunnel: [w428 w432] -> w306
                tunnel: w365 -> [w429 w431]
                tunnel: w340 -> [_ w430]
                tunnel: w321 -> [w428 _]
                tunnel: w320 -> [w427 _]
                frame False {
                }
                frame True {
                  n149 = call "next_move.vi"("Snake In"=w431, "Snake Unit"=w430, "Direction"=w435, "Direction max"=w436) -> ("Y"=w432:i32, "X"=w433:i32, "Snake Out"=w434:T22)  [unwired: 5 in]
                }
              }
              n150 = Round To Nearest(number=w351) -> (nearest integer value=w350:dbl)
              n151 = Wait (ms)(milliseconds to wait=w350) -> ()  [unwired: 1 out]
              n152 = local read "direction2"() -> (w348:dbl)
              n153 = call "collision_self.vi"("Snake Plot"=w308) -> ("Result"=w370:bool)  [unwired: 10 in]
              n154 = call "collision_wall.vi"("World Size"=w303, "Y"=w306, "X"=w307) -> ("Result"=w369:bool)  [unwired: 7 in]
              n155 = call "resolve_apples.vi"("Y"=w306, "X"=w307, "Max Apples"="Max Apples", "Apple Unit"=w340, "World Size"=w303, "Apples In"=w335) -> ("Ate Apple"=w360:bool, "Apples Out"=w328:T22)  [unwired: 4 in]
              n156 = Or(x=w370, y=w369) -> (x .or. y?=w315:bool)
              n157 = Select(t=w358, s=w360, f=w359) -> (s? t:f=w313:i32)
              "Score 1" <- w313
              n158 = Select(t=w332, s=w360, f=w364) -> (s? t:f=w361:i32)
              n159 = Subtract(x=w332, y=w361) -> (x-y=w363:i32)
              n160 = Less?(x=w363, y=w362) -> (x < y?=w344:bool)
              n161 = case shown="False" w296 {
                tunnel: w349 -> [_ w426]
                tunnel: w348 -> [_ w425]
                tunnel: w347 -> [w419 w424]
                tunnel: [w419 w423] -> w305
                tunnel: [w418 w422] -> w302
                tunnel: [w417 w421] -> w318
                tunnel: w340 -> [_ w420]
                tunnel: w319 -> [w418 _]
                tunnel: w291 -> [w417 _]
                frame False {
                }
                frame True {
                  n162 = call "next_move.vi"("Snake In"=w424, "Snake Unit"=w420, "Direction"=w425, "Direction max"=w426) -> ("Y"=w421:i32, "X"=w422:i32, "Snake Out"=w423:T22)  [unwired: 5 in]
                }
              }
              n163 = call "collision_self.vi"("Snake Plot"=w305) -> ("Result"=w343:bool)  [unwired: 10 in]
              n164 = Unbundle By Name(w305) -> ("X"=w304:i32[], "Y"=w301:i32[])
              n165 = call "collision_wall.vi"("World Size"=w303, "Y"=w318, "X"=w302) -> ("Result"=w342:bool)  [unwired: 7 in]
              n166 = call "resolve_apples.vi"("Y"=w318, "X"=w302, "Max Apples"="Max Apples", "Apple Unit"=w340, "World Size"=w303, "Apples In"=w328) -> ("Ate Apple"=w339:bool, "Apples Out"=w325:T22)  [unwired: 4 in]
              n167 = Or(x=w343, y=w342) -> (x .or. y?=w314:bool)
              n168 = Select(t=w338, s=w339, f=w337) -> (s? t:f=w312:i32)
              "Score 2" <- w312
              n169 = Select(t=w332, s=w339, f=w336) -> (s? t:f=w333:i32)
              n170 = case shown="True" w298 {
                tunnel: w308 -> [_ w396]
                tunnel: w307 -> [_ w393]
                tunnel: w306 -> [_ w392]
                tunnel: w304 -> [_ w391]
                tunnel: w303 -> [_ _]
                tunnel: w302 -> [_ w390]
                tunnel: w301 -> [_ w389]
                tunnel: [w373 w383] -> w293
                tunnel: [w376 w385] -> w295
                tunnel: w297 -> [w375 _]
                tunnel: w296 -> [w372 _]
                tunnel: w294 -> [w377 w388]
                tunnel: w292 -> [w374 w387]
                tunnel: w291 -> [_ w382]
                frame False {
                  n171 = case shown="True" w374 {
                    selector: w374 -> [_ w379]
                    tunnel: [w378 w379] -> w373
                    tunnel: w372 -> [w378 _]
                    frame False {
                    }
                    frame True {
                    }
                  }
                  n172 = case shown="True" w377 {
                    tunnel: [w380 w381] -> w376
                    tunnel: w377 -> [_ w381]
                    tunnel: w375 -> [w380 _]
                    frame False {
                    }
                    frame True {
                    }
                  }
                }
                frame True {
                  n173 = Unbundle By Name(w396) -> ("X"=w395:i32[], "Y"=w394:i32[])
                  n174 = call "ResolveCollisonWithOther.vi"("Snake 1 X's"=w395, "Snake1X"=w393, "Snake2X"=w390, "Snake1Y"=w392, "Snake 1 Y's"=w394, "Snake 2 Y's"=w389, "Snake 2 X's"=w391, "Snake2Y"=w382) -> ("Snake 1 Died"=w386:bool, "Snake 2 Died"=w384:bool)  [unwired: 18 in]
                  n175 = case shown="False" w388 {
                    selector: w388 -> [_ w400]
                    tunnel: [w399 w400] -> w385
                    tunnel: w386 -> [w399 _]
                    frame False {
                    }
                    frame True {
                    }
                  }
                  n176 = case shown="False" w387 {
                    selector: w387 -> [_ w398]
                    tunnel: w384 -> [w397 _]
                    tunnel: [w397 w398] -> w383
                    frame False {
                    }
                    frame True {
                    }
                  }
                }
              }
              n177 = case shown="False" w344 {
                tunnel: [w444 w445] -> w326
                tunnel: w371 -> [w443 _]
                tunnel: w308 -> [w442 w445]
                frame False {
                  n178 = call "xyplot_delete.vi"("index"=w443, "XY Plot Input"=w442) -> ("XY Plot Output"=w444:T22)  [unwired: 9 in]
                }
                frame True {
                }
              }
              n179 = Subtract(x=w332, y=w333) -> (x-y=w331:i32)
              n180 = Less?(x=w331, y=w330) -> (x < y?=w329:bool)
              n181 = Or(x=w293, y=w314) -> (x .or. y?=w300:bool)
              n182 = Or(x=w295, y=w315) -> (x .or. y?=w299:bool)
              n183 = local read "Add To Score"() -> (w309:bool)
              n184 = Not(x=w299) -> (.not. x?=w323:bool)
              n185 = And(x=w299, y=w300) -> (x .and. y?=w341:bool)
              n186 = Not(x=w300) -> (.not. x?=w322:bool)
              n187 = Exclusive Or(1:w300, 2:w299) -> (0:w317:bool)
              n188 = case shown="False" w329 {
                tunnel: [w439 w440] -> w327
                tunnel: w345 -> [w438 _]
                tunnel: w305 -> [w437 w440]
                frame False {
                  n189 = call "xyplot_delete.vi"("index"=w438, "XY Plot Input"=w437) -> ("XY Plot Output"=w439:T22)  [unwired: 9 in]
                }
                frame True {
                }
              }
              n190 = local read "Done"() -> (w355:bool)
              n191 = And(x=w317, y=w309) -> (x .and. y?=w316:bool)
              n192 = case shown="True" w316 {
                tunnel: w299 -> [_ w408]
                tunnel: w313 -> [w402 w407]
                tunnel: w312 -> [w401 w406]
                tunnel: [w402 w403] -> w311
                tunnel: [w401 w404] -> w310
                frame False {
                  (unwired) TRUE
                }
                frame True {
                  n193 = case shown="False" w408 {
                    tunnel: w407 -> [w409 w416]
                    tunnel: w406 -> [w412 w414]
                    tunnel: [w410 w414] -> w404
                    tunnel: [w409 w413] -> w403
                    frame True {
                      n194 = Add(x=w412, y=2) -> (x+y=w410:i32)
                    }
                    frame False {
                      n195 = Add(x=w416, y=2) -> (x+y=w413:i32)
                    }
                  }
                  n196 = local write "Add To Score"(FALSE) -> ()
                }
              }
              n197 = local read "Done"() -> (w356:bool)
              n198 = Or(x=w355, y=w341) -> (x .or. y?=w354:bool)
              n199 = Build Array(w326, w327, w325) -> (w324:T22[])
              n200 = Not(x=w356) -> (.not. x?=w357:bool)
              n201 = case shown="True" w357 {
                tunnel: w324 -> [_ w441]
                frame False {
                }
                frame True {
                  "XY Graph" <- w441
                }
              }
            }
          }
          frame #1 {
            # "Game Over"
            n202 = Wait (ms)(milliseconds to wait=u32 3000) -> ()  [unwired: 1 out]
          }
        }
        n203 = Random Number (0-1)() -> (number: 0 to 1=w266:dbl)
        n204 = Multiply(x=w266, y=w252) -> (x*y=w269:dbl)
        n205 = Round Toward -Infinity(1:w269) -> (0:w256:dbl)
        "direction1" <- w256
        n206 = Add(x=2.0, y=w256) -> (x+y=w242:dbl)
        n207 = Less?(x=w242, y=4.0) -> (x < y?=w243:bool)
        n208 = Subtract(x=w242, y=4.0) -> (x-y=w241:dbl)
        n209 = Select(t=w242, s=w243, f=w241) -> (s? t:f=→"direction2":dbl)
      }
      n210 = while {
        stop <- FALSE stop-if-true
        # "Hide Snake when Enabled."
        n211 = Wait Until Next ms Multiple(millisecond multiple=u32 10) -> ()  [unwired: 1 out]
        n212 = local read "Status"() -> (w196:T1)
        n213 = Not Equal?(x=w196, y=T1."Enabled" ("Status")) -> (x != y?=w194:bool)
        n214 = Not(x="Force Hide Snake") -> (.not. x?=w192:bool)
        n215 = control-ref of="XY Graph"() -> (w197:refnum<vi>)
        n216 = And(x=w194, y=w192) -> (x .and. y?=w191:bool)
        n217 = property class="XYGraph (strict)"(reference=w197, "Visible"=w191) -> ()  [unwired: 1 in, 2 out]
      }
    }
  }
